vi "Launch timer test.vi"   [LabVIEW 2015, in "Timer test.lvclass"]
uses:
  Timer test.lvclass
  Mag Lab Root/Mag Lab Root.lvclass/Mag Lab Root.ctl
  <vilib>/ActorFramework/Message Enqueuer/Message Enqueuer.lvclass/Message Enqueuer.ctl
  <vilib>/ActorFramework/Message Enqueuer/Enqueue.vi
  <vilib>/ActorFramework/Message Priority Queue/Priority Enqueue.vi
  Mag Lab Root Messages/Open Front Panel Msg/Open Front Panel Msg.lvclass
  <vilib>/ActorFramework/Actor/Actor.lvclass
  <vilib>/ActorFramework/Stop Msg/Stop Msg.lvclass
  Mag Lab Root/Mag Lab Root.lvclass
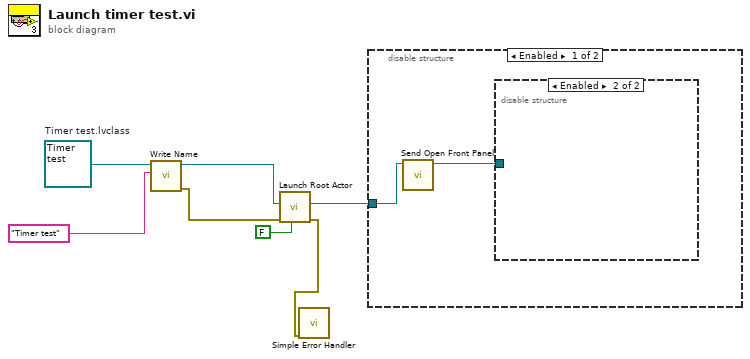
[diagram p0: block diagram]
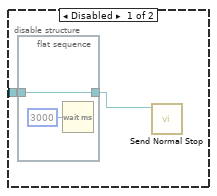
[diagram p2: hidden frame]
diagram:
  w7 = refnum<class "Timer test.lvclass"> refnum  # Timer test.lvclass
  n1 = call "Write Name.vi"("Name"="Timer test" ("Requestor"), "Mag Lab Root in"=w7) -> ("error out"=w1:errorcluster, "Mag Lab Root out"=w3:refnum<class "Timer test.lvclass">)  [unwired: 8 in]
  n2 = call <vilib>:"Launch Root Actor.vi"("Open Actor Core front panel? (F)"=FALSE, "error in (no error)"=w1, "Actor"=w3) -> ("error out"=w4:errorcluster, "Actor's Enqueuer"=w6:refnum<class "Message Enqueuer.lvclass">)  [unwired: 7 in]
  n3 = call <vilib>:"Simple Error Handler.vi"("error in (no error)"=w4) -> ()  [unwired: 4 in, 5 out]
  n4 = disable-structure shown="Enabled" {
    disable-tunnel: w6 -> [w9 _]
    frame Enabled {
      n5 = call "Send Open Front Panel.vi"("Message Enqueuer"=w9) -> ("Message Enqueuer out"=w8:refnum<class "Message Enqueuer.lvclass">)  [unwired: 9 in, 1 out]
      n6 = disable-structure shown="Enabled" {
        disable-tunnel: w8 -> [w11 _]
        frame Disabled {
          n7 = flat-sequence {
            tunnel: w11 -> [w12]
            tunnel: [w12] -> w10
            frame #0 {
              n8 = Wait (ms)(milliseconds to wait=u32 3000) -> ()  [unwired: 1 out]
            }
          }
          n9 = call <vilib>:"Send Normal Stop.vi"("Message Enqueuer"=w10) -> ()  [unwired: 10 in, 1 out]
        }
        frame Enabled {
        }
      }
    }
    frame Disabled {
    }
  }
